vi "Extract Exceptions.vi"(11 "Message":u8[](array[numeric]) format="%.0x") -> (2 "Exception":bool, 3 "Display string":string)   [LabVIEW 2015, in "VC940.lvlib"]
uses:
  VC940.lvlib
panel:
  out "Low":bool
  out "Off":bool
  out "Overload":bool
  out "U64":u64 format="%.0x"
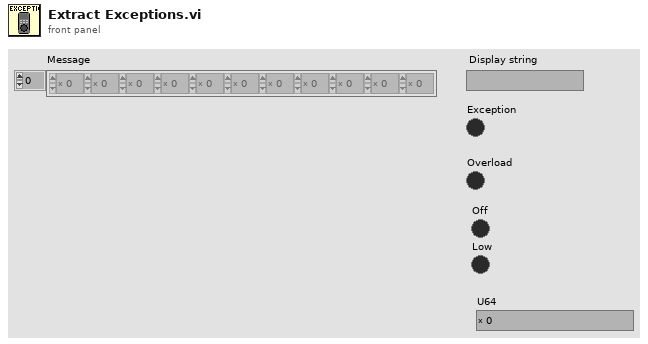
[diagram p1: front panel]
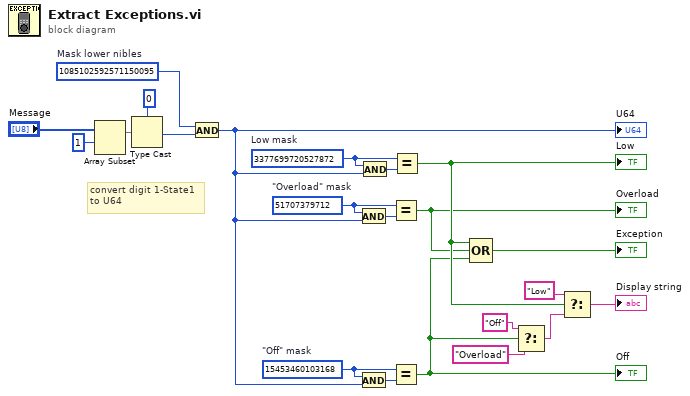
[diagram p0: block diagram]
diagram:
  w6 = u64 15453460103168  # "Off" mask
  w7 = u64 51707379712  # "Overload" mask
  w22 = u64 3377699720527872  # Low mask
  w18 = u64 1085102592571150095  # Mask lower nibles
  # "convert digit 1-State1\nto U64"
  n1 = Array Subset(array="Message", index=1) -> (w14:u8[])  [unwired: 1 in]
  n2 = Type Cast(type=u64 0 ("index"), x=w14) -> (*(type *) &x=w17:u64)
  n3 = And(x=w18, y=w17) -> (x .and. y?=w4:u64)
  "U64" <- w4
  n4 = And(x=w7, y=w4) -> (x .and. y?=w8:u64)
  n5 = And(x=w6, y=w4) -> (x .and. y?=w5:u64)
  n6 = And(x=w22, y=w4) -> (x .and. y?=w19:u64)
  n7 = Equal?(x=w7, y=w8) -> (x = y?=w2:bool)
  "Overload" <- w2
  n8 = Equal?(x=w6, y=w5) -> (x = y?=w1:bool)
  "Off" <- w1
  n9 = Equal?(x=w22, y=w19) -> (x = y?=w3:bool)
  "Low" <- w3
  n10 = Compound Arithmetic op=OR(w3, w2, w1) -> (→"Exception":bool)
  n11 = Select(t="Off" ("String 2"), s=w1, f="Overload" ("String 2")) -> (s? t:f=w10:string)
  n12 = Select(t="Low" ("String 2"), s=w3, f=w10) -> (s? t:f=→"Display string":string)
